vi "ParseAllBlocksMessages.vi"(0 "Path":path) -> (1 "SCM2CA Msg Cluster Array":cluster{"Names":string[], "Codes":i32[]}, 2 "VM INP from SCM Msg Cluster Array":cluster{"Names":string[], "Codes":i32[]}, 3 "SCM2VM Msg Cluster Array":cluster{"Names":string[], "Codes":i32[]}, 4 "VM2GUI Msg Cluster Array":cluster{"Names":string[], "Codes":i32[]}, 5 "VM2SCM Msg Cluster Array":cluster{"Names":string[], "Codes":i32[]}, 6 "SCM2VP Msg Cluster Array":cluster{"Names":string[], "Codes":i32[]}, 7 "CA2GUI Msg Cluster Array":cluster{"Names":string[], "Codes":i32[]}, 8 "SCM2VP Msg Cluster Array":cluster{"Names":string[], "Codes":i32[]}, 9 "COM2CA MSG Cluster Array":cluster{"Names":string[], "Codes":i32[]})   [LabVIEW 2010]
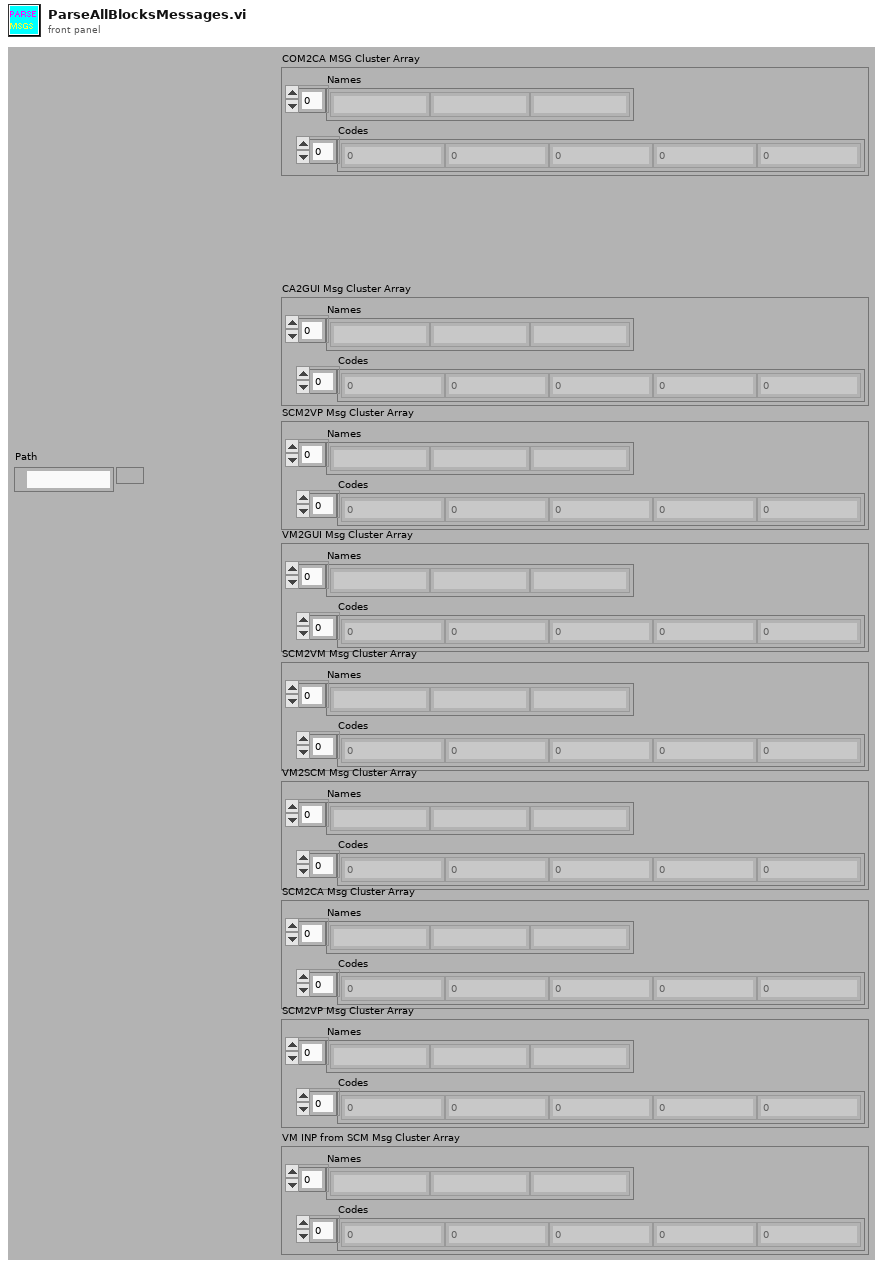
[diagram p1: front panel]
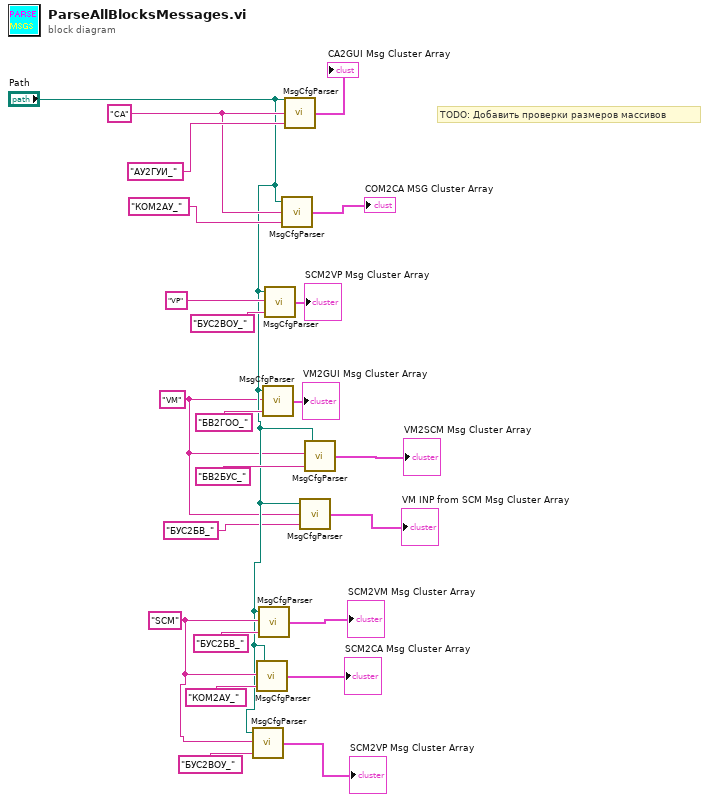
[diagram p0: block diagram]
diagram:
  w11 = "SCM" ("name or relative path")
  w3 = "VM" ("name or relative path")
  w20 = "CA" ("name or relative path")
  # "TODO: Добавить проверки размеров массивов"
  n1 = call "MsgCfgParser.vi"("search string"="БУС2ВОУ_", "name or relative path"=w11, "stripped path"="Path") -> ("Msg Cluster Array"=→"SCM2VP Msg Cluster Array":cluster{"Names":string[], "Codes":i32[]})
  n2 = call "MsgCfgParser.vi"("search string"="КОМ2АУ_", "name or relative path"=w11, "stripped path"="Path") -> ("Msg Cluster Array"=→"SCM2CA Msg Cluster Array":cluster{"Names":string[], "Codes":i32[]})
  n3 = call "MsgCfgParser.vi"("search string"="БУС2БВ_", "name or relative path"=w11, "stripped path"="Path") -> ("Msg Cluster Array"=→"SCM2VM Msg Cluster Array":cluster{"Names":string[], "Codes":i32[]})
  n4 = call "MsgCfgParser.vi"("search string"="БВ2ГОО_", "name or relative path"=w3, "stripped path"="Path") -> ("Msg Cluster Array"=→"VM2GUI Msg Cluster Array":cluster{"Names":string[], "Codes":i32[]})
  n5 = call "MsgCfgParser.vi"("search string"="БУС2ВОУ_", "name or relative path"="VP", "stripped path"="Path") -> ("Msg Cluster Array"=→"SCM2VP Msg Cluster Array":cluster{"Names":string[], "Codes":i32[]})
  n6 = call "MsgCfgParser.vi"("search string"="КОМ2АУ_" ("name or relative path"), "name or relative path"=w20, "stripped path"="Path") -> ("Msg Cluster Array"=→"COM2CA MSG Cluster Array":cluster{"Names":string[], "Codes":i32[]})
  n7 = call "MsgCfgParser.vi"("search string"="АУ2ГУИ_" ("name or relative path"), "name or relative path"=w20, "stripped path"="Path") -> ("Msg Cluster Array"=→"CA2GUI Msg Cluster Array":cluster{"Names":string[], "Codes":i32[]})
  n8 = call "MsgCfgParser.vi"("search string"="БУС2БВ_", "name or relative path"=w3, "stripped path"="Path") -> ("Msg Cluster Array"=→"VM INP from SCM Msg Cluster Array":cluster{"Names":string[], "Codes":i32[]})
  n9 = call "MsgCfgParser.vi"("search string"="БВ2БУС_", "name or relative path"=w3, "stripped path"="Path") -> ("Msg Cluster Array"=→"VM2SCM Msg Cluster Array":cluster{"Names":string[], "Codes":i32[]})
